vi "color2bit_array.vi"(11 "Input Color":i32) -> (3 "Bit Array":u8[](array[numeric]))   [LabVIEW 2013]
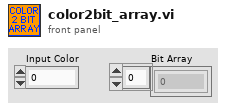
[diagram p1: front panel]
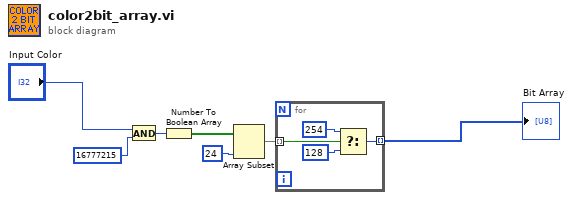
[diagram p0: block diagram]
diagram:
  n1 = And(x="Input Color", y=16777215) -> (x .and. y?=w4:i32)
  n2 = Number To Boolean Array(number=w4) -> (Boolean array=w5:bool[])
  n3 = Array Subset(array=w5, length=24) -> (w6:bool[])  [unwired: 1 in]
  n4 = for {
    tunnel: w6 -> [w11] mode=indexing
    tunnel: [w8] -> w1 mode=indexing
    n5 = Select(t=u8 254, s=w11, f=u8 128 ("t")) -> (s? t:f=w8:u8)
  }
  "Bit Array" <- w1
